vi "Generate DAC data.vi"(2 "End time":dbl format="%.2f", 3 "Default voltages":dbl[](array[numeric]) format="%.2f", 4 "Input Array":T1(array[cluster]) {"Voltages" format="%.2f"; "Times" format="%.2f"}) -> (0 "times":dbl[](array[numeric]), 1 "Output":dbl[][](array[numeric]) format="%.2f")   [LabVIEW 2017]
doc: "This vi creates an array of voltages to be programmed into the static DAQ's buffer. If the channel is not enabled, then it is set to the default voltage. \n The inputs are a terminating time, an array of default voltages, an array of ending voltages, and an array of clusters containing voltages, times, an enable boolean, the number of hinge points.\n The output is a 2-D array of voltages where each collumn corresponds to a different DAQ channel."
uses:
  globals/RIO and DAC defaults global.vi
panel:
  # "Note: The PCI 6733 DAQ card outputs the first row of voltages immediately after being\nprogrammed and then ignores the first trigger pulse. In order to get the card to behave\nas needed, the first row of the array is padded with the default voltages. Extra trigger pulses\nhave been added into pick module.vi for the extra values in the array. Currently the first trigger\nis hard coded to an absolute time of 100 us in 'pick module.vi'. After that time the card is ready to be triggered\nto whatever voltages the user desires."
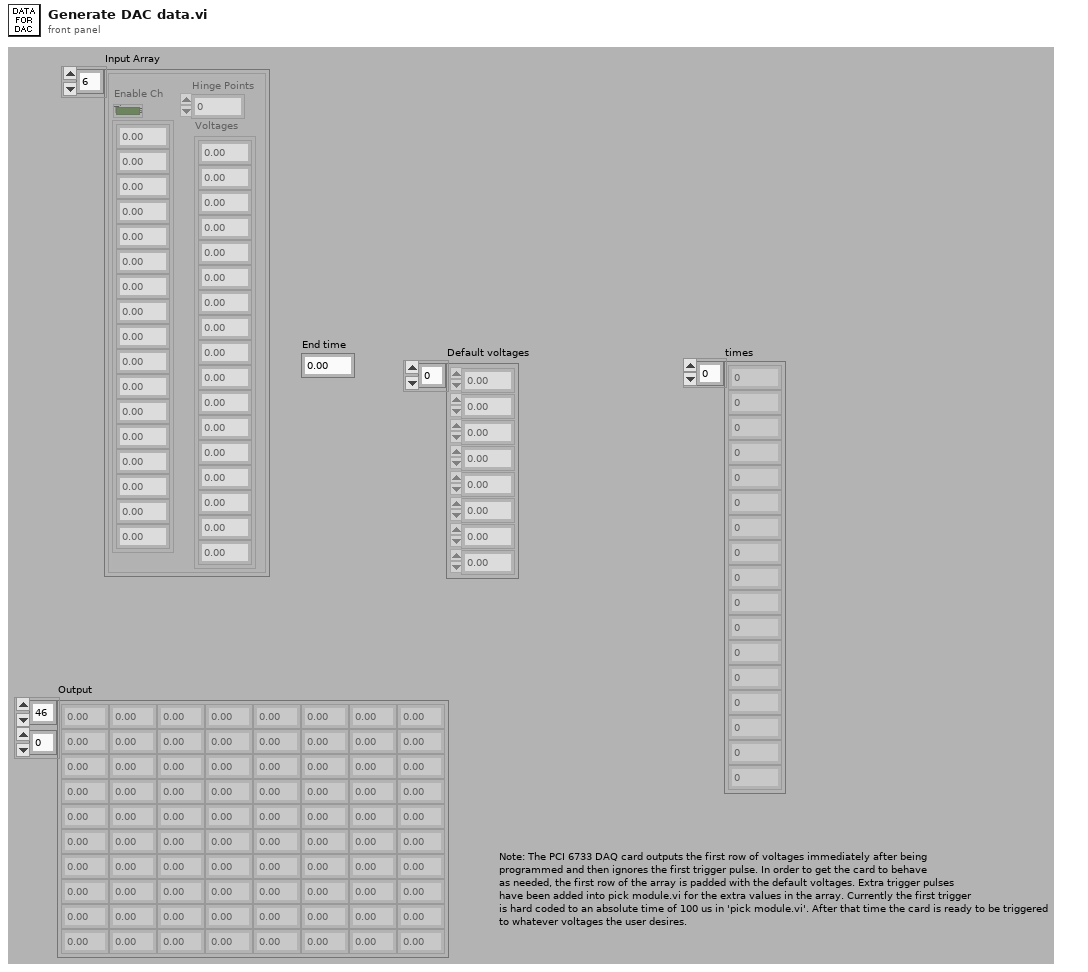
[diagram p1: front panel]
types:
  T1 = cluster{"Times":dbl[], "Voltages":dbl[], "Enable Ch":bool, "Hinge Points":u8}[]
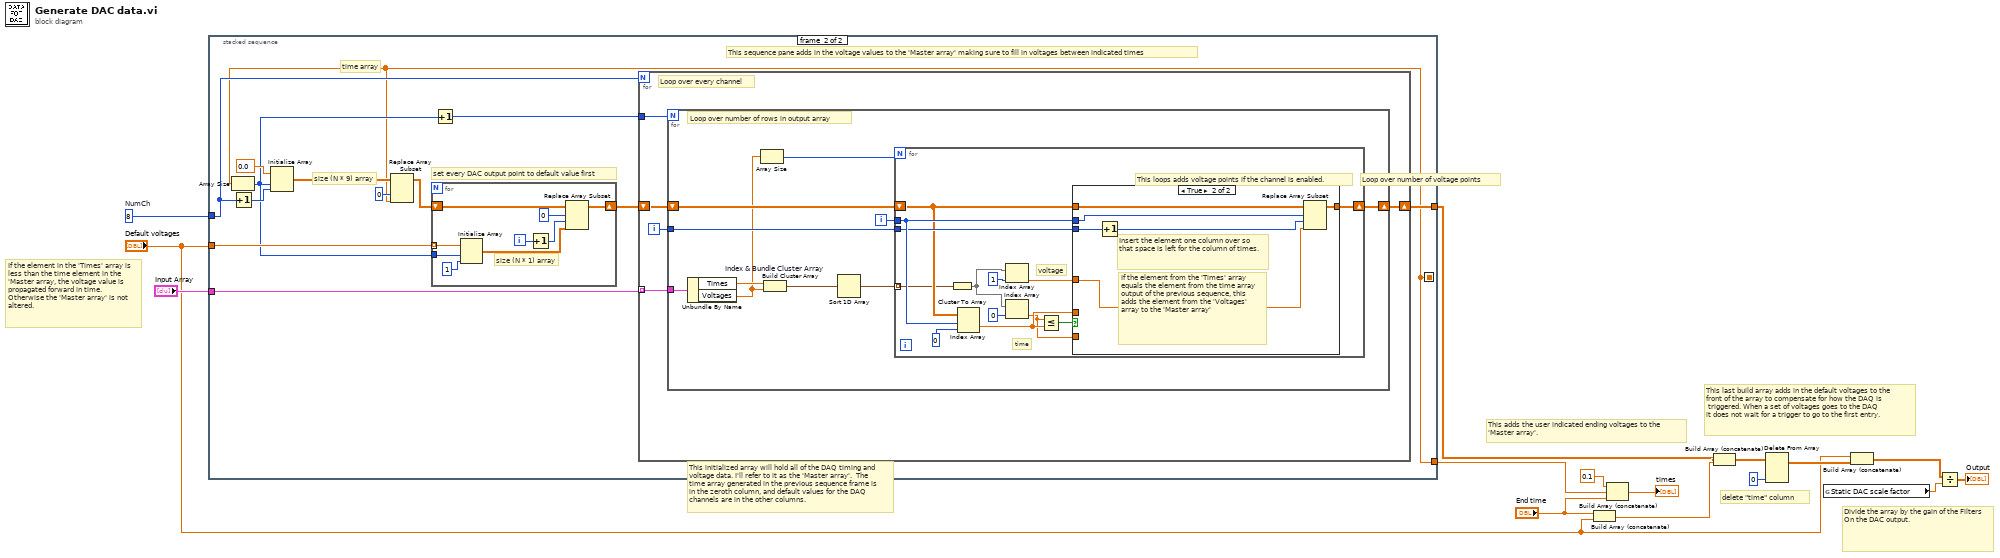
[diagram p0: block diagram]
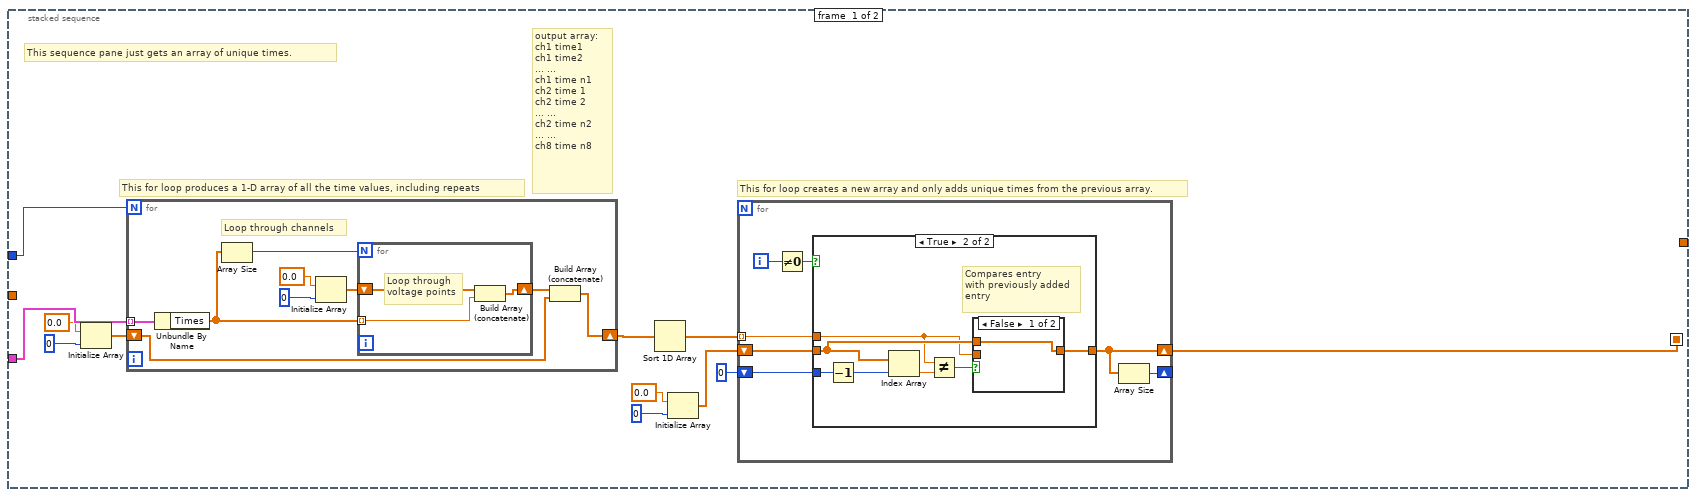
[diagram p2: hidden frame]
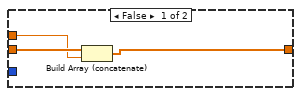
[diagram p3: hidden frame]
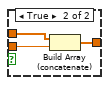
[diagram p4: hidden frame]
diagram:
  w15 = 8  # NumCh
  # "delete \"time\" column"
  # "If the element in the 'Times' array is less than the time element in the 'Master array, the voltage value is propagated forward in time. Otherwise the 'Master array' is not altered."
  # "Divide the array by the gain of the Filters\nOn the DAC output."
  # "This last build array adds in the default voltages to the \nfront of the array to compensate for how the DAQ is\n triggered. When a set of voltages goes to the DAQ\nit does not wait for a trigger to go to the first entry."
  # "This adds the user indicated ending voltages to the \n'Master array'."
  n1 = stacked-sequence {
    seq-local: [w17 _] -> [_ w61]
    tunnel: "Input Array" -> [w27 w73]
    tunnel: w15 -> [w18 w66]
    tunnel: [_ w72] -> w9
    tunnel: "Default voltages" -> [_ w65]
    tunnel: [_ w61] -> w5
    frame #0 {
      # "output array:\nch1 time1\nch1 time2\n... ...\nch1 time n1\nch2 time 1\nch2 time 2\n... ...\nch2 time n2\n... ...\nch8 time n8"
      # "This sequence pane just gets an array of unique times."
      # "This for loop creates a new array and only adds unique times from the previous array."
      # "This for loop produces a 1-D array of all the time values, including repeats"
      n2 = Initialize Array(0.0 ("Element Data"), 0 ("Dimension Size")) -> (w25:dbl[])
      n3 = for {
        N: w18 -> [_]
        tunnel: w27 -> [w57] mode=indexing
        shift-right: [w55] -> w23
        shift-left: w25 -> [w56]
        # "Loop through channels"
        n4 = Unbundle By Name(w57) -> ("Times"=w54:dbl[])
        n5 = Array Size(array=w54) -> (size(s)=w49:i32)
        n6 = Initialize Array(0.0 ("Element Data"), 0 ("Dimension Size")) -> (w51:dbl[])
        n7 = for {
          N: w49 -> [_]
          tunnel: w54 -> [w58] mode=indexing
          shift-right: [w59] -> w50
          shift-left: w51 -> [w60]
          # "Loop through \nvoltage points"
          n8 = Build Array (concatenate)(w60, w58) -> (w59:dbl[])
        }
        n9 = Build Array (concatenate)(w50, w56) -> (w55:dbl[])
      }
      n10 = Sort 1D Array(array=w23) -> (sorted array=w22:dbl[])
      n11 = Initialize Array(0.0 ("Element Data"), 0 ("Dimension Size")) -> (w19:dbl[])
      n12 = for {
        tunnel: w22 -> [w32] mode=indexing
        shift-right: [w31] -> w17
        shift-left: w19 -> [w33]
        shift-right: [w30] -> _
        shift-left: 0 -> [w28]
        i -> [w29]
        n13 = Not Equal To 0?(x=w29) -> (x != 0?=w34:bool)
        n14 = case shown="True" w34 {
          tunnel: w33 -> [w37 w40]
          tunnel: w32 -> [w36 w39]
          tunnel: [w35 w38] -> w31
          tunnel: w28 -> [_ w42]
          frame False {
            n15 = Build Array (concatenate)(w37, w36) -> (w35:dbl[])
          }
          frame True {
            # "Compares entry \nwith previously added\nentry"
            n16 = Decrement(x=w42) -> (x-1=w41:i32)
            n17 = Index Array(array=w40, index=w41) -> (element=w43:dbl)
            n18 = Not Equal?(x=w39, y=w43) -> (x != y?=w44:bool)
            n19 = case shown="False" w44 {
              tunnel: w40 -> [w45 w48]
              tunnel: w39 -> [_ w47]
              tunnel: [w45 w46] -> w38
              frame False {
              }
              frame True {
                n20 = Build Array (concatenate)(w48, w47) -> (w46:dbl[])
              }
            }
          }
        }
        n21 = Array Size(array=w31) -> (size(s)=w30:i32)
      }
    }
    frame #1 {
      # "size (N * 9) array"
      # "time array"
      # "set every DAC output point to default value first"
      # "This initialized array will hold all of the DAQ timing and voltage data. I'll refer to it as the 'Master array'.  The time array generated in the previous sequence frame is in the zeroth column, and default values for the DAQ channels are in the other columns."
      # "This sequence pane adds in the voltage values to the 'Master array' making sure to fill in voltages between indicated times"
      n22 = Array Size(array=w61) -> (size(s)=w62:i32)
      n23 = Increment(x=w66) -> (x+1=w67:i32)
      n24 = Initialize Array(0.0 ("Element Data"), w62, w67) -> (w71:dbl[][])
      n25 = Replace Array Subset(array=w71, new element=w61, index (col)=0 ("Index (row)")) -> (w64:dbl[][])  [unwired: 1 in]
      n26 = for {
        tunnel: w65 -> [w79] mode=indexing
        shift-right: [w74] -> w63
        shift-left: w64 -> [w81]
        tunnel: w62 -> [w78]
        i -> [w82]
        # "size (N * 1) array"
        n27 = Initialize Array(w79, w78, 1 ("dimension size")) -> (w75:dbl[][])
        n28 = Increment(x=w82) -> (x+1=w80:i32)
        n29 = Replace Array Subset(array=w81, new element=w75, index (row)=0 ("disabled index (row)"), index (col)=w80) -> (w74:dbl[][])
      }
      n30 = Increment(x=w62) -> (x+1=w70:i32)
      n31 = for {
        N: w66 -> [_]
        tunnel: w73 -> [w87] mode=indexing
        tunnel: w70 -> [w86]
        shift-right: [w83] -> w72
        shift-left: w63 -> [w84]
        i -> [w85]
        # "Loop over every channel"
        n32 = for {
          N: w86 -> [_]
          tunnel: w87 -> [w97]
          tunnel: w85 -> [w95]
          shift-right: [w93] -> w83
          shift-left: w84 -> [w94]
          i -> [w96]
          # "Loop over number of rows in output array"
          n33 = Unbundle By Name(w97) -> ("Times"=w92:dbl[], "Voltages"=w89:dbl[])
          n34 = Array Size(array=w89) -> (size(s)=w88:i32)
          n35 = Build Cluster Array "Index & Bundle Cluster Array"(w92, w89) -> (w91:cluster{"Numeric":dbl, "Numeric":dbl}[])
          n36 = Sort 1D Array(array=w91) -> (sorted array=w90:cluster{"Numeric":dbl, "Numeric":dbl}[])
          n37 = for {
            N: w88 -> [_]
            tunnel: w96 -> [w108]
            tunnel: w95 -> [w107]
            shift-right: [w104] -> w93
            shift-left: w94 -> [w105]
            tunnel: w90 -> [w103] mode=indexing
            # "time"
            # "voltage"
            # "This loops adds voltage points if the channel is enabled."
            # "Loop over number of voltage points"
            n38 = Cluster To Array(cluster=w103) -> (array=w102:dbl[])
            n39 = Index Array(array=w105, index (row)=w108, index (col)=0 ("Disabled Index (col)")) -> (element=w106:dbl)
            n40 = Index Array(array=w102, index=1) -> (element=w99:dbl)
            n41 = Index Array(array=w102, index=0) -> (element=w98:dbl)
            n42 = Less Or Equal?(x=w98, y=w106) -> (x <= y?=w110:bool)
            n43 = case shown="True" w110 {
              tunnel: w105 -> [w111 w114]
              tunnel: w99 -> [_ w112]
              tunnel: w108 -> [_ w117]
              tunnel: w107 -> [_ w116]
              tunnel: [w111 w113] -> w104
              tunnel: w106 -> [_ _]
              tunnel: w98 -> [_ _]
              frame False {
              }
              frame True {
                # "Insert the element one column over so that space is left for the column of times."
                # "If the element from the 'Times' array equals the element from the time array output of the previous sequence, this adds the element from the 'Voltages' array to the 'Master array'"
                n44 = Increment(x=w116) -> (x+1=w115:i32)
                n45 = Replace Array Subset(array=w114, new element=w112, index (row)=w117, index (col)=w115) -> (w113:dbl[][])
              }
            }
          }
        }
      }
    }
  }
  n46 = Build Array (concatenate)("End time", "Default voltages") -> (w13:dbl[])
  n47 = Build Array (concatenate)(0.1 ("Index (row)"), w5, "End time") -> (→"times":dbl[])
  n48 = Build Array (concatenate)(w9, w13) -> (w12:dbl[][])
  n49 = Delete From Array(array=w12, index (col)=0 ("Disabled Index (col)")) -> (array with subset deleted=w10:dbl[][])  [unwired: 2 in, 1 out]
  n50 = global read "RIO and DAC defaults global.vi" "Static DAC scale factor"() -> (w1:dbl)
  n51 = Build Array (concatenate)("Default voltages", w10) -> (w8:dbl[][])
  n52 = Divide(x=w8, y=w1) -> (x/y=→"Output":dbl[][])
